vi "p2_Control_nivel.vi"() -> ()   [LabVIEW 2019]
panel:
  in  "Accion":bool
  in  "Llenado/\nVaciado":bool
  in  "Velocidad":bool
  out "Tanque\nVacio":bool
  out "Tanque\nLleno":bool
  out "Paro":bool
  out "Llenando":bool
  out "Vaciando":bool
  out "Tanque":dbl(slide) scale=0.0..1000.0
  # "Alta"
  # "Baja"
  # "Continuar"
  # "Parar"
  # "Llenar"
  # "Vaciar"
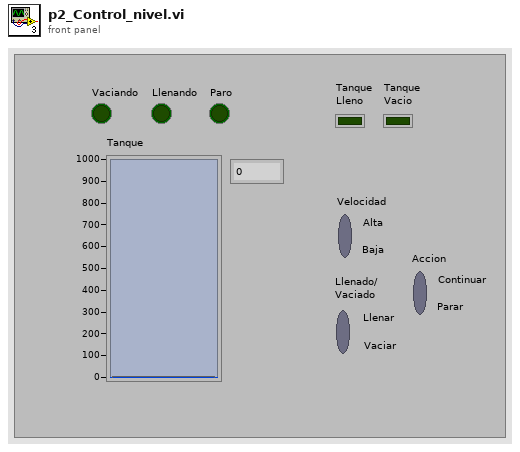
[diagram p1: front panel]
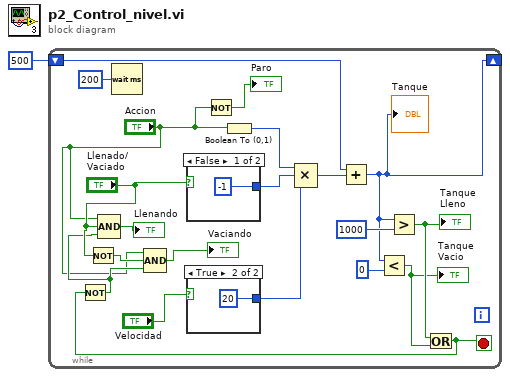
[diagram p0: block diagram]
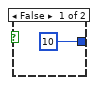
[diagram p2: hidden frame]
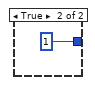
[diagram p3: hidden frame]
diagram:
  n1 = while {
    shift-right: [w5] -> _
    shift-left: 500 -> [w14]
    stop <- w11 stop-if-true
    n2 = Not(x="Llenado/\nVaciado") -> (.not. x?=w4:bool)
    n3 = Wait (ms)(milliseconds to wait=u32 200) -> ()  [unwired: 1 out]
    n4 = case shown="False" "Llenado/\nVaciado" {
      tunnel: [-1 1] -> w18
      frame False {
      }
      frame True {
      }
    }
    n5 = case shown="True" "Velocidad" {
      tunnel: [10 20] -> w17
      frame False {
      }
      frame True {
      }
    }
    n6 = Not(x="Accion") -> (.not. x?=→"Paro":bool)
    n7 = Boolean To (0,1)(Boolean="Accion") -> (0, 1=w19:i16)
    n8 = Compound Arithmetic op=MULTIPLY(w19, w18, w17) -> (w15:i32)
    n9 = Add(x=w14, y=w15) -> (x+y=w5:i32)
    "Tanque" <- w5
    n10 = Less?(x=w5, y=i16 0 ("x")) -> (x < y?=w12:bool)
    "Tanque\nVacio" <- w12
    n11 = Greater?(x=w5, y=u16 1000) -> (0:w13:bool)
    "Tanque\nLleno" <- w13
    n12 = Or(x=w13, y=w12) -> (x .or. y?=w11:bool)
    n13 = Not(x=w11) -> (.not. x?=w3:bool)
    n14 = Compound Arithmetic op=AND("Accion", "Llenado/\nVaciado", w3) -> (→"Llenando":bool)
    n15 = Compound Arithmetic op=AND("Accion", w4, w3) -> (→"Vaciando":bool)
  }
